vi "Mindsensors NXTCam Config.vi"(10 "Node Data":T1, 11 "NXT":T2) -> ()   [LabVIEW 2010]
uses:
  <vilib>/NXT/Subs/LVHSConnector.ctl
  Datatypes/Node.ctl
  UI Controls/PlugInControls/Pluginbackground.ctl
  <vilib>/Utility/miscctls.llb/LVPointTypeDef.ctl
  <vilib>/NXT/Block Support/HWPage.SensorMode.ctl
  <vilib>/NXT/Block Support/HWPage.SensorType.ctl
  ConvertNodeAddrSensor.vi
panel:
  out "NXT Port":i32
  in  "Go / Stop Button":bool
  in  "stoploop":i32
  out "Color":u8
  out "# of Objects Found":u8
  out "Loop Status":string
  out "Xtl":u8
  out "Ytl":u8
  out "Xbr":u8
  out "Ybr":u8
  out "# of Objects\n found":u8
  out "Color":u8
  out "Tracks the First Object it Finds":picture
  in  "Device Address":u8=2 format="%x"
  in  "Sensor Parameters":string
  in  "Name":string
  out "Headline":string="Type (auto populated)"
  in  "Instance Specific Data":cluster{"Example Data":dbl}
  in  "Reset":bool
  in  "Save":bool
  in  "Stop":bool
  out "Background":T3=TRUE
  # "<- No controls below this line"
  # "Common controls such as Buttons, Rings, Sliders, Graphs, Decorations, etc can be found in the <labview>\\Targets\\NI\\NXT\\NXT Toolkit\\Schematic Editor\\UI Controls\\Plugin Controls\\ folder. Use these controls when possible to ensure a consistent look and feel with LabVIEW Education Edition."
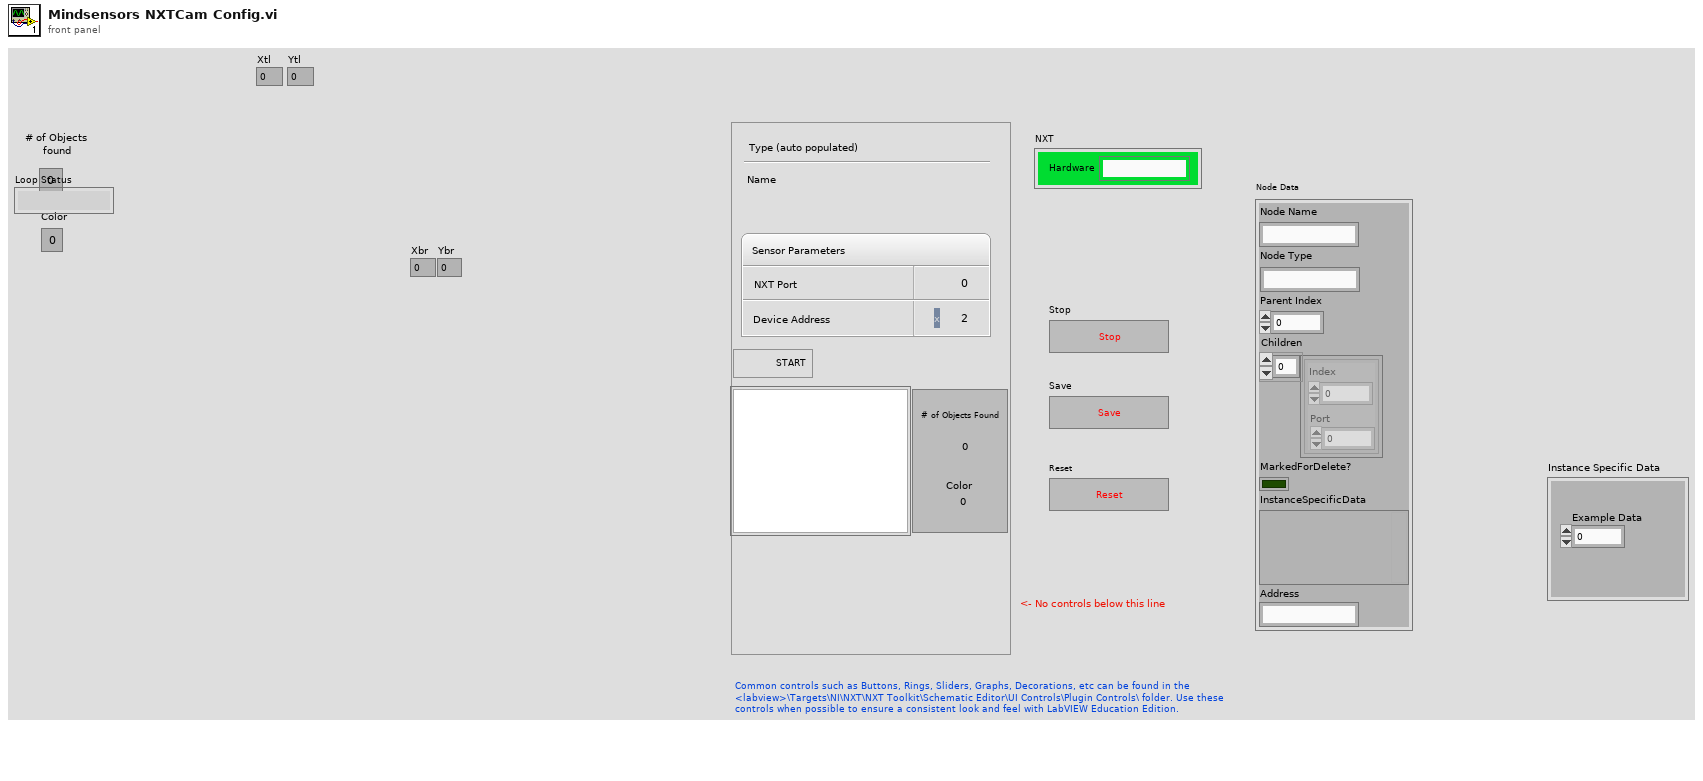
[diagram p1: front panel]
types:
  T1 = typedef "Node.ctl" = cluster{"Node Name":string, "Node Type":string, "Parent Index":i16, "Children":cluster{"Index":u16, "Port":u16}[], "MarkedForDelete?":bool, "InstanceSpecificData":variant, "Address":string}
  T2 = typedef "LVHSConnector.ctl" = cluster{"Hardware":string, "Flattened String":string}
  T3 = typedef "Pluginbackground.ctl" = bool
  T4 = typedef "LVPointTypeDef.ctl" = cluster{"Horizontal":i16, "Vertical":i16}
  T5 = cluster{"Width":i16, "Style":enum32{"Solid", "Dash", "Dot", "DashDot", "DashDotDot"}}
  T6 = typedef "HWPage.SensorMode.ctl" = u8
  T7 = typedef "HWPage.SensorType.ctl" = u8
  T8 = typedef "NXT_InputPort.ctl" = u8
  T9 = typedef "nxt.ctl" = cluster{"nxtHandle":u32, "fileHandle":u32, "fileIterHandle":u32, "moduleHandle":u32, "modIterHandle":u32, "nxtIterHandle":u32}
  T10 = enum8{"Enabled", "Disabled", "Disabled and Grayed Out"}
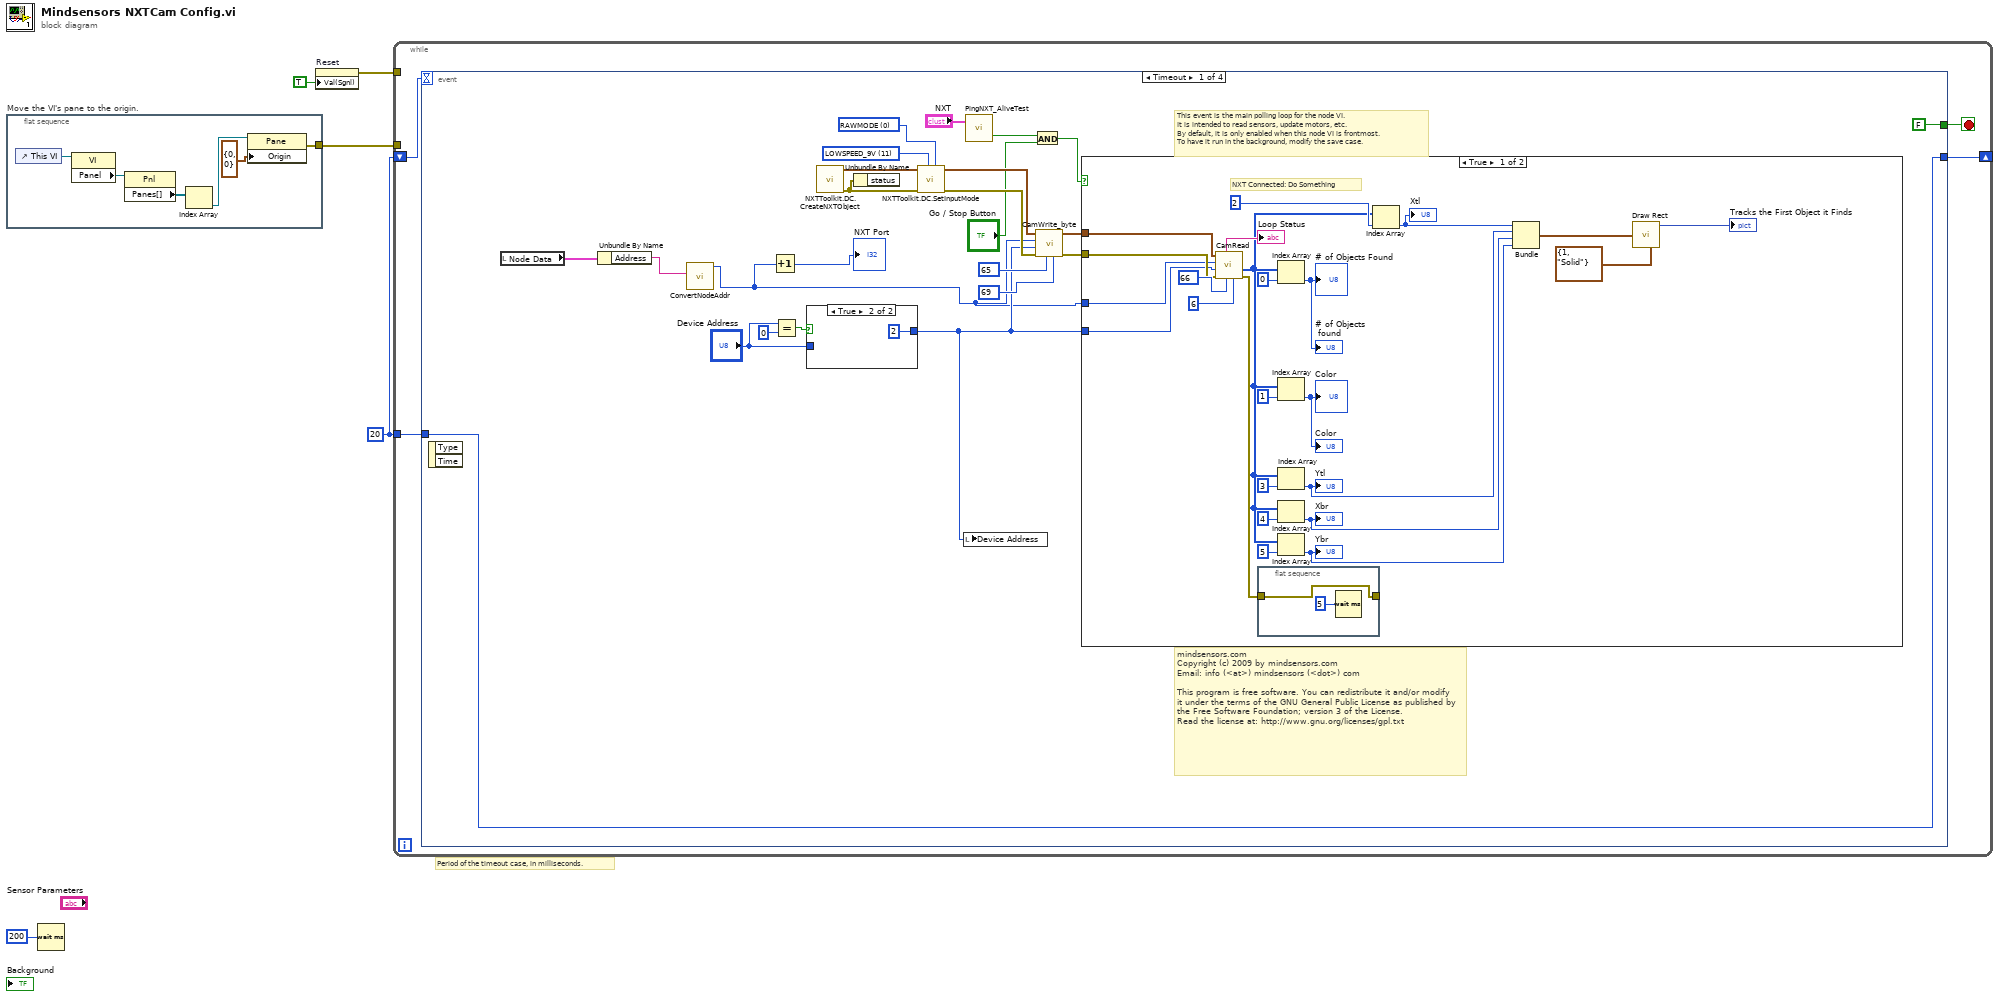
[diagram p0: block diagram]
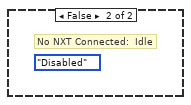
[diagram p3: hidden frame]
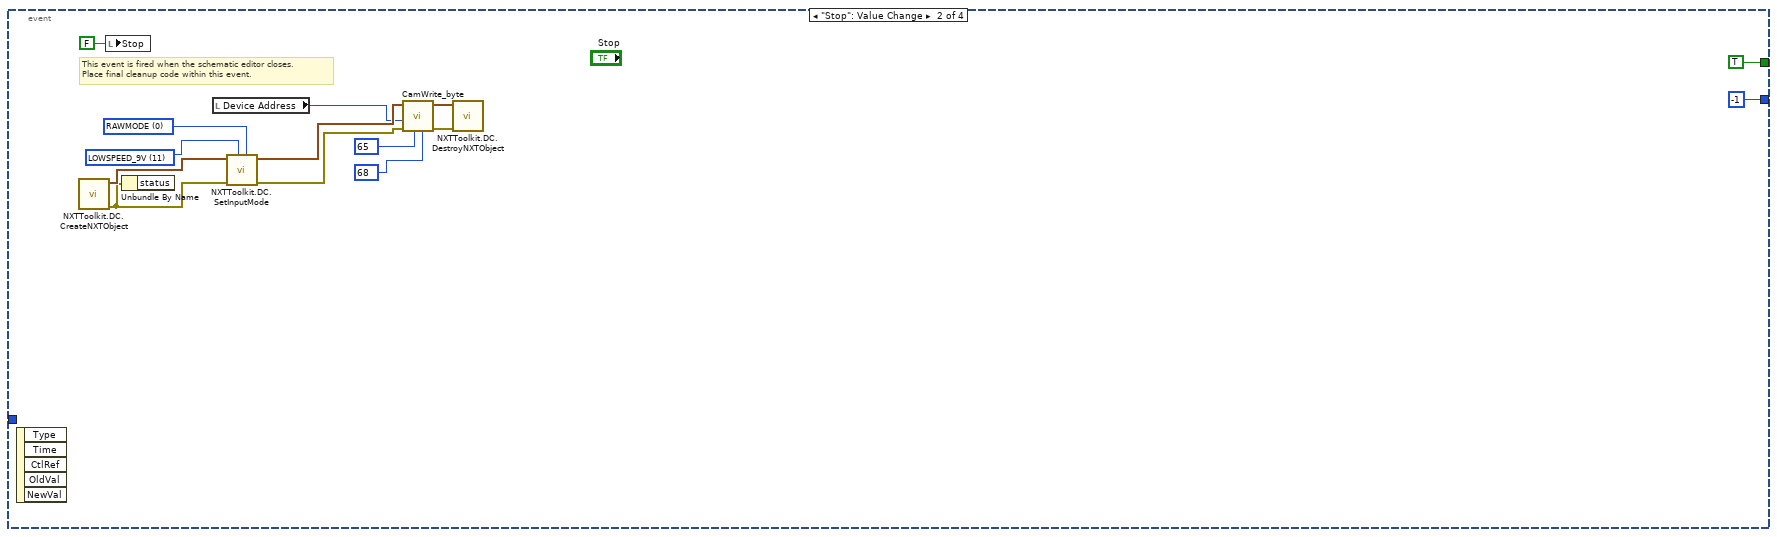
[diagram p4: hidden frame]
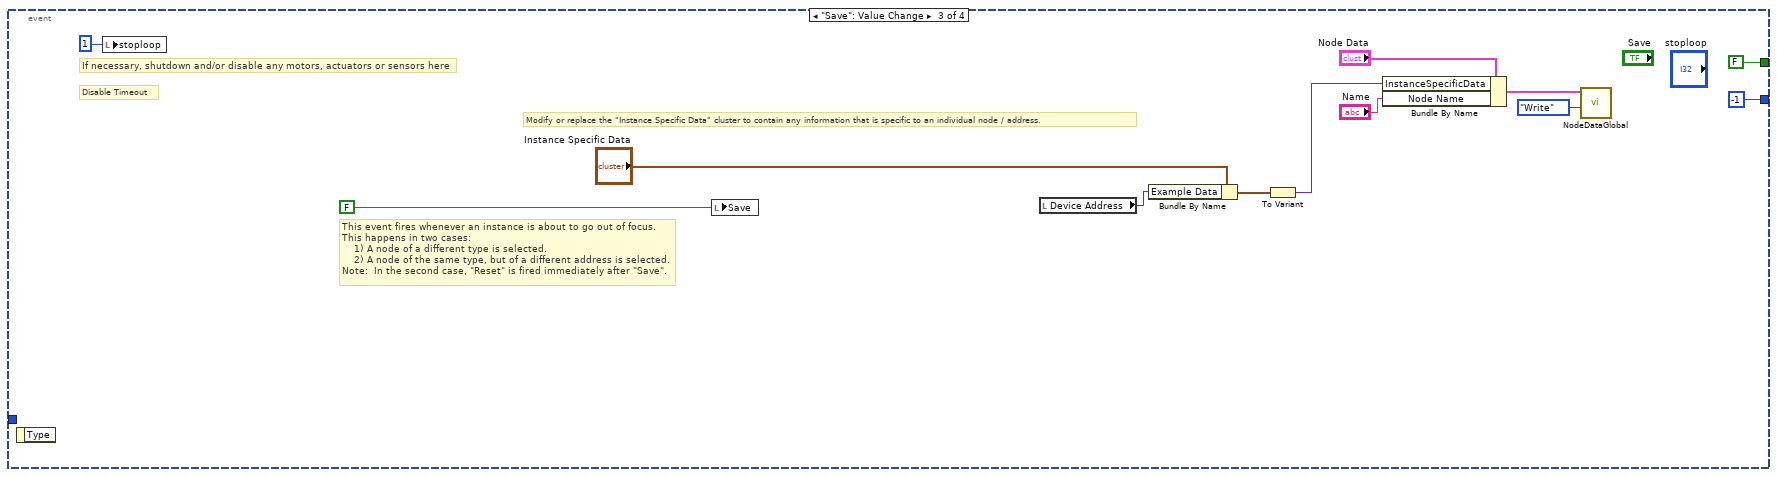
[diagram p5: hidden frame]
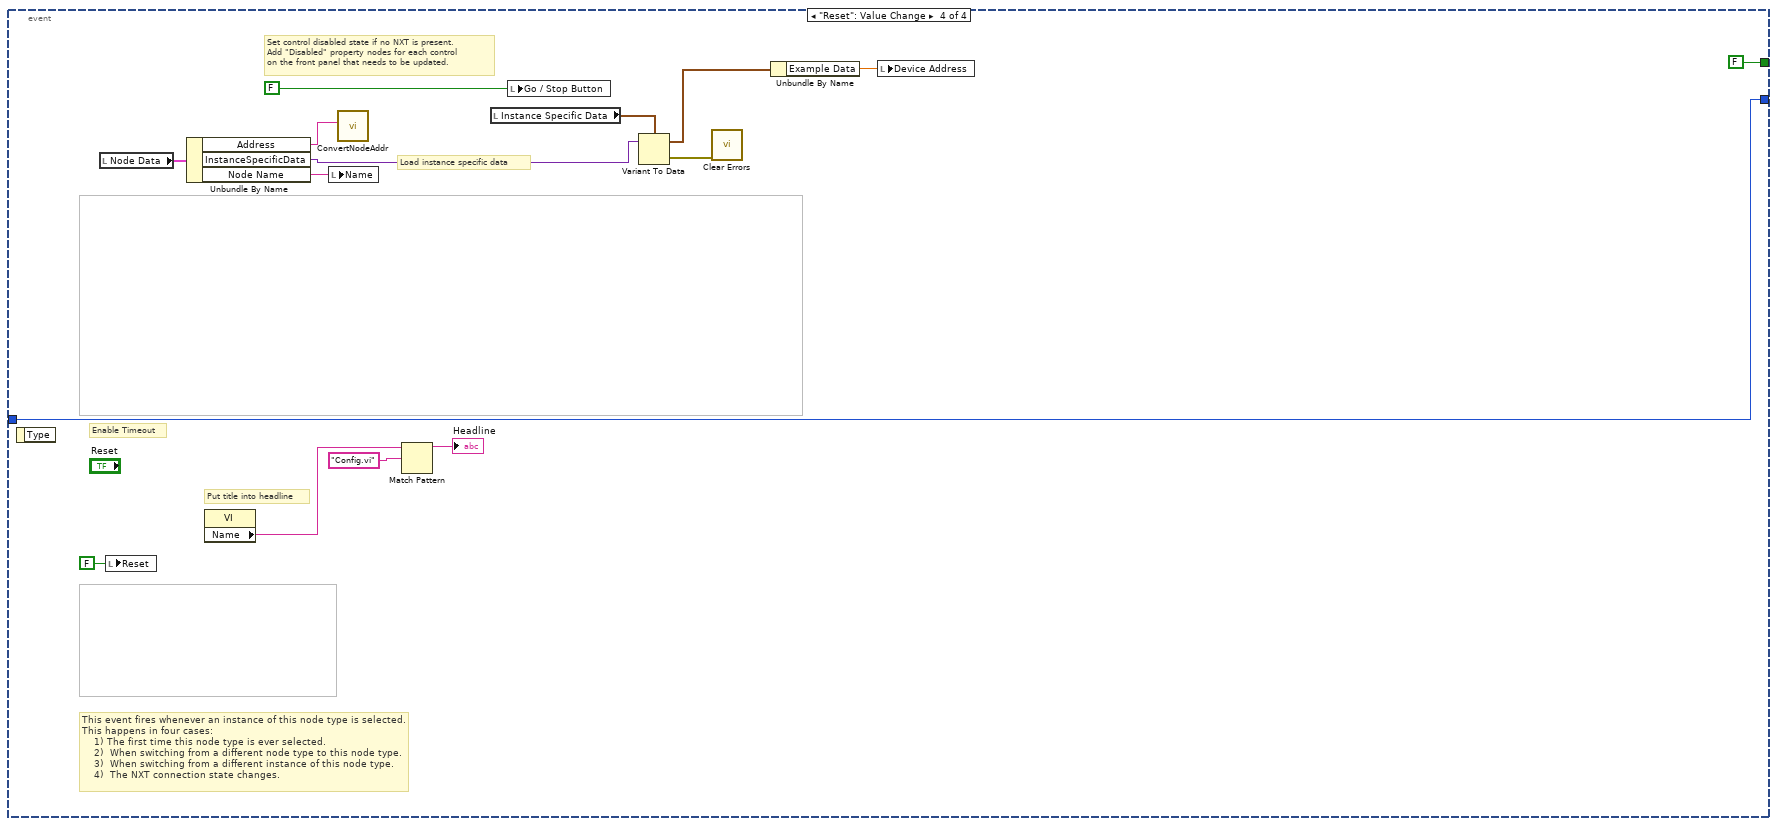
[diagram p6: hidden frame]
diagram:
  w3 = 20
  # "Period of the timeout case, in milliseconds."
  n1 = flat-sequence "Move the VI's pane to the origin." {
    tunnel: [w6] -> w2
    frame #0 {
      n2 = control-ref of="This VI"() -> (w7:refnum<vi>)
      n3 = property class="VI"(reference=w7) -> ("Panel"=w8:refnum<vi>)  [unwired: 1 in, 2 out]
      n4 = property class="Pnl"(reference=w8) -> ("Panes[]"=w9:refnum<vi>[])  [unwired: 1 in, 2 out]
      n5 = Index Array(array=w9) -> (element=w10:refnum<vi>)  [unwired: 1 in]
      n6 = property class="Pane"(reference=w10, "Origin"=T4 {"Horizontal"=0, "Vertical"=0}) -> (error out=w6:errorcluster)  [unwired: 1 in, 1 out]
    }
  }
  n7 = Wait (ms)(milliseconds to wait=u32 200) -> ()  [unwired: 1 out]
  n8 = property on="Reset" class="Bool (strict)"("Val(Sgnl)"=TRUE ("Value (Signaling)")) -> (error out=w4:errorcluster)  [unwired: 2 in, 1 out]
  n9 = while {
    tunnel: w4 -> [_]
    shift-right: [w13] -> _
    shift-left: w3 -> [w14]
    tunnel: w3 -> [w12]
    tunnel: w2 -> [_]
    stop <- w15 stop-if-true
    n10 = event shown="[0] Timeout" {
      selector: _ -> [_ _ _ _]
      dyn-events: _ -> [_ _ _ _]
      timeout: w14 -> [_ _ _ _]
      tunnel: [FALSE TRUE FALSE FALSE] -> w15
      tunnel: [w39 -1 -1 w104] -> w13
      tunnel: w12 -> [w39 _ _ w104]
      event Timeout {
        w36 = T6 0 items=["RAWMODE"=0, "BOOLEANMODE"=32, "TRANSITIONCNTMODE"=64, "PERIODCOUNTERMODE"=96, "PCTFULLSCALEMODE"=128, "CELSIUSMODE"=160, "FAHRENHEITMODE"=192, "ANGLESTEPMODE"=224] ("Sensor Mode (RAWMODE)")
        w35 = T7 11 items=["NO_SENSOR", "SWITCH", "TEMPERATURE", "REFLECTION", "ANGLE", "LIGHT_ACTIVE", "LIGHT_INACTIVE", "SOUND_DB", "SOUND_DBA", "CUSTOM", "LOWSPEED", "LOWSPEED_9V", "HIGHSPEED"] ("Sensor Type (NO_SENSOR)")
        # "mindsensors.com\nCopyright (c) 2009 by mindsensors.com\nEmail: info (<at>) mindsensors (<dot>) com\n\nThis program is free software. You can redistribute it and/or modify\nit under the terms of the GNU General Public License as published by\nthe Free Software Foundation; version 3 of the License.\nRead the license at: http://www.gnu.org/licenses/gpl.txt"
        # "This event is the main polling loop for the node VI.\nIt is intended to read sensors, update motors, etc.\nBy default, it is only enabled when this node VI is frontmost.\nTo have it run in the background, modify the save case."
        n11 = event-data() -> ()  [unwired: 1 in, 2 out]
        n12 = local read "Node Data"() -> (w37:T1)
        n13 = Unbundle By Name(w37) -> ("Address"=w18:string)
        n14 = call-poly "ConvertNodeAddr.vi"("Sensor Port"=w18) -> ("NXT Port"=w17:T8)  [unwired: 6 in, 4 out]
        n15 = Increment(x=w17) -> (x+1=→"NXT Port":T8)
        n16 = Equal?(x="Device Address", y=u8 0) -> (x = y?=w21:bool)
        n17 = case shown="True" w21 {
          tunnel: [w40 u8 2 ("Device Addr 2")] -> w19
          tunnel: "Device Address" -> [w40 _]
          frame False {
          }
          frame True {
          }
        }
        n18 = call <vilib>:"NXTToolkit.DC.CreateNXTObject.vi"() -> ("error out"=w33:errorcluster, "NXTObject"=w34:T9)  [unwired: 9 in, 1 out]
        n19 = Unbundle By Name(w33) -> ()  [unwired: 1 out]
        n20 = call <vilib>:"NXTToolkit.DC.SetInputMode.vi"("Sensor Mode (RAWMODE)"=w36, "Sensor Type (NO_SENSOR)"=w35, "error in (no error)"=w33, "NXTObject"=w34) -> ("error out"=w28:errorcluster, "NXTObject dup"=w29:T9)  [unwired: 5 in, 1 out]
        n21 = local write "Device Address"(w19) -> ()
        n22 = call <vilib>:"PingNXT_AliveTest.vi"("NXT"="NXT") -> ("connected?"=w25:bool)  [unwired: 1 in, 1 out]
        n23 = And(x=w25, y="Go / Stop Button") -> (x .and. y?=w23:bool)
        n24 = call <vilib>:"CamWrite_byte.vi"("Data byte"=u8 69, "Reg Address"=u8 65, "error in (no error)"=w28, "Device Address"=w19, "Input Port in"=w17, "NXTObject"=w29) -> ("error out"=w26:errorcluster, "NXTObject dup"=w27:T9)  [unwired: 1 in, 3 out]
        n25 = case shown="True" w23 {
          tunnel: w17 -> [w43 _]
          tunnel: w27 -> [w45 _]
          tunnel: w26 -> [w44 _]
          tunnel: w19 -> [w42 _]
          frame True {
            # "NXT Connected: Do Something"
            n26 = call <vilib>:"CamRead.vi"("bytes to read"=u8 6, "Reg Address"=u8 66, "error in (no error)"=w44, "Device Address"=w42, "Input Port in"=w43, "NXTObject"=w45) -> ("error out"=w48:errorcluster, "data Buffer"=w50:u8[], "string"=→"Loop Status":string)  [unwired: 3 out]
            n27 = flat-sequence {
              tunnel: [w66] -> _
              tunnel: w48 -> [w66]
              frame #0 {
                n28 = Wait (ms)(milliseconds to wait=u32 5) -> ()  [unwired: 1 out]
              }
            }
            n29 = Index Array(array=w50, index=0) -> (element=→"# of Objects\n found" →"# of Objects Found":u8)
            n30 = Index Array(array=w50, index=1) -> (element=→"Color" →"Color":u8)
            n31 = Index Array(array=w50, index=3) -> (element=w53:u8)
            "Ytl" <- w53
            n32 = Index Array(array=w50, index=4) -> (element=w52:u8)
            "Xbr" <- w52
            n33 = Index Array(array=w50, index=5) -> (element=w51:u8)
            "Ybr" <- w51
            n34 = Index Array(array=w50, index=2) -> (element=w55:u8)
            "Xtl" <- w55
            n35 = Bundle(w55, w53, w52, w51) -> (w56:cluster{u8, u8, u8, u8})  [unwired: 1 in]
            n36 = call <vilib>:"Draw Rect.vi"("rect"=w56, "pen"=T5 {"Width"=1, "Style"=enum."Solid"}) -> ("new picture"=→"Tracks the First Object it Finds":picture)  [unwired: 7 in]
          }
          frame False {
            (unwired) T10."Disabled" ("Disabled")
            # "No NXT Connected:  Idle"
          }
        }
      }
      event "Stop": Value Change {
        w78 = T6 0 items=["RAWMODE"=0, "BOOLEANMODE"=32, "TRANSITIONCNTMODE"=64, "PERIODCOUNTERMODE"=96, "PCTFULLSCALEMODE"=128, "CELSIUSMODE"=160, "FAHRENHEITMODE"=192, "ANGLESTEPMODE"=224] ("Sensor Mode (RAWMODE)")
        w77 = T7 11 items=["NO_SENSOR", "SWITCH", "TEMPERATURE", "REFLECTION", "ANGLE", "LIGHT_ACTIVE", "LIGHT_INACTIVE", "SOUND_DB", "SOUND_DBA", "CUSTOM", "LOWSPEED", "LOWSPEED_9V", "HIGHSPEED"] ("Sensor Type (NO_SENSOR)")
        # "This event is fired when the schematic editor closes.\nPlace final cleanup code within this event."
        n37 = event-data() -> ()  [unwired: 1 in, 5 out]
        n38 = call <vilib>:"NXTToolkit.DC.CreateNXTObject.vi"() -> ("error out"=w75:errorcluster, "NXTObject"=w76:T9)  [unwired: 9 in, 1 out]
        n39 = local write "Stop"(FALSE ("stop")) -> ()
        n40 = Unbundle By Name(w75) -> ()  [unwired: 1 out]
        n41 = local read "Device Address"() -> (w68:u8)
        n42 = call <vilib>:"NXTToolkit.DC.SetInputMode.vi"("Sensor Mode (RAWMODE)"=w78, "Sensor Type (NO_SENSOR)"=w77, "error in (no error)"=w75, "NXTObject"=w76) -> ("error out"=w69:errorcluster, "NXTObject dup"=w70:T9)  [unwired: 5 in, 1 out]
        n43 = call <vilib>:"CamWrite_byte.vi"("Data byte"=68, "Reg Address"=u8 65, "error in (no error)"=w69, "Device Address"=w68, "NXTObject"=w70) -> ("error out"=w71:errorcluster, "NXTObject dup"=w72:T9)  [unwired: 2 in, 3 out]
        n44 = call <vilib>:"NXTToolkit.DC.DestroyNXTObject.vi"("error in (no error)"=w71, "NXTObject"=w72) -> ()  [unwired: 9 in, 1 out]
      }
      event "Save": Value Change {
        # "If necessary, shutdown and/or disable any motors, actuators or sensors here"
        # "Modify or replace the \"Instance Specific Data\" cluster to contain any information that is specific to an individual node / address."
        # "Disable Timeout"
        # "This event fires whenever an instance is about to go out of focus.\nThis happens in two cases:\n    1) A node of a different type is selected.\n    2) A node of the same type, but of a different address is selected.\nNote:  In the second case, \"Reset\" is fired immediately after \"Save\"."
        n45 = event-data() -> ()  [unwired: 1 in, 1 out]
        n46 = local write "stoploop"(1 ("stoploop")) -> ()
        n47 = local write "Save"(FALSE ("stop")) -> ()
        n48 = local read "Device Address"() -> (w83:u8)
        n49 = Bundle By Name(cluster="Instance Specific Data", "Example Data"=w83) -> (w84:cluster{"Example Data":dbl})
        n50 = To Variant(anything=w84) -> (Variant=w91:variant)
        n51 = Bundle By Name(cluster="Node Data", "InstanceSpecificData"=w91, "Node Name"="Name") -> (w90:T1)
        n52 = call "NodeDataGlobal.vi"("Action"=enum16{"Read", "Write"}."Write", "Node Data In"=w90) -> ()  [unwired: 8 in, 2 out]
      }
      event "Reset": Value Change {
        # "Set control disabled state if no NXT is present.\nAdd \"Disabled\" property nodes for each control\non the front panel that needs to be updated."
        # "Load instance specific data"
        # "Enable Timeout"
        # "This event fires whenever an instance of this node type is selected.\nThis happens in four cases:\n    1) The first time this node type is ever selected.\n    2)  When switching from a different node type to this node type.\n    3)  When switching from a different instance of this node type. \n    4)  The NXT connection state changes."
        # "Put title into headline"
        n53 = event-data() -> ()  [unwired: 1 in, 1 out]
        n54 = local read "Node Data"() -> (w105:T1)
        n55 = local write "Reset"(FALSE ("Reset")) -> ()
        n56 = Unbundle By Name(w105) -> ("Address"=w96:string, "InstanceSpecificData"=w106:variant, "Node Name"=w98:string)
        n57 = property class="VI"() -> ("Name"=w100:string)  [unwired: 2 in, 2 out]
        n58 = local write "Name"(w98) -> ()
        n59 = call-poly "ConvertNodeAddr.vi"("Sensor Port"=w96) -> ()  [unwired: 6 in, 5 out]
        n60 = Match Pattern(string=w100, regular expression="Config.vi") -> (before substring=→"Headline":string)  [unwired: 1 in, 3 out]
        n61 = local read "Instance Specific Data"() -> (w103:cluster{"Example Data":dbl})
        n62 = local write "Go / Stop Button"(FALSE ("Go / Stop Button")) -> ()
        n63 = Variant To Data(Variant=w106, type=w103) -> (error out=w102:errorcluster, data=w97:cluster{"Example Data":dbl})  [unwired: 1 in]
        n64 = call <vilib>:"Clear Errors.vi"("error in (no error)"=w102) -> ()  [unwired: 6 in, 1 out]
        n65 = Unbundle By Name(w97) -> ("Example Data"=w95:dbl)
        n66 = local write "Device Address"(w95) -> ()
      }
    }
  }
